vi "Write to JSON File.vi"(8 "error in (no error)":errorcluster, 10 "JSON String":string, 11 "Byte Stream File in":refnum<file>) -> (0 "error out":errorcluster)   [LabVIEW 2020, in "JSON File Manipulation.lvlib"]
doc: "Reformats the JSON string in a pretty format and writes it to the JSON file, replacing all previous content."
uses:
  JSON File Manipulation.lvlib
  <vilib>/JDP Science/JSONtext/JSONtext.lvlib
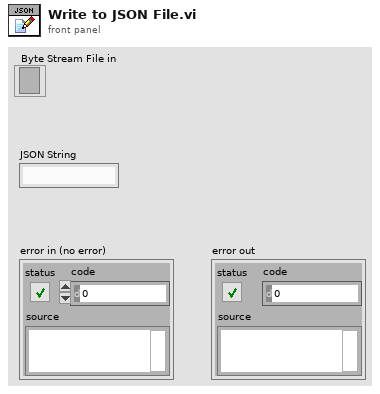
[diagram p1: front panel]
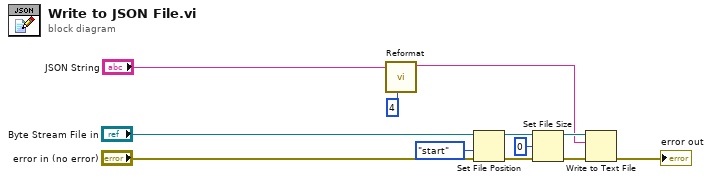
[diagram p0: block diagram]
diagram:
  n1 = call <vilib>:"Reformat.vi"("Pretty Print Levels"=4, "JSON"="JSON String") -> ("<JSON>First JSON Value\n\n<JSON>"=w1:string)  [unwired: 6 in, 3 out]
  n2 = Set File Position(refnum="Byte Stream File in", from (0:start)=enum16{"start", "end", "current"}."start", error in="error in (no error)") -> (refnum out=w9:refnum<file>, error out=w7:errorcluster)  [unwired: 1 in]
  n3 = Set File Size(4:w7, 6:i64 0 ("size (in bytes)"), 7:w9) -> (0:w8:errorcluster, 3:w10:refnum<file>)
  n4 = Write to Text File(file (use dialog)=w10, text=w1, error in=w8) -> (error out=→"error out":errorcluster)  [unwired: 1 in, 2 out]
